vi "find fit -- normalize complex culture.vi"(11 "z in window":cdb[](array[numeric])) -> (0 "z  normalized":cdb[](array[numeric]), 1 "normalization factor":dbl=1.0, 2 "data center":cdb, 3 "# of elements":i32)   [LabVIEW 2021]
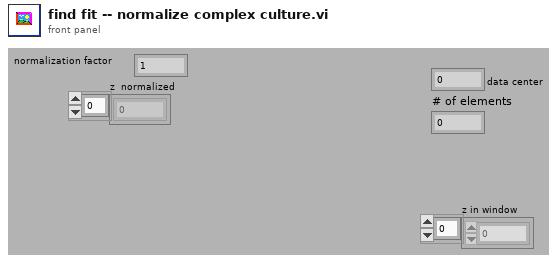
[diagram p1: front panel]
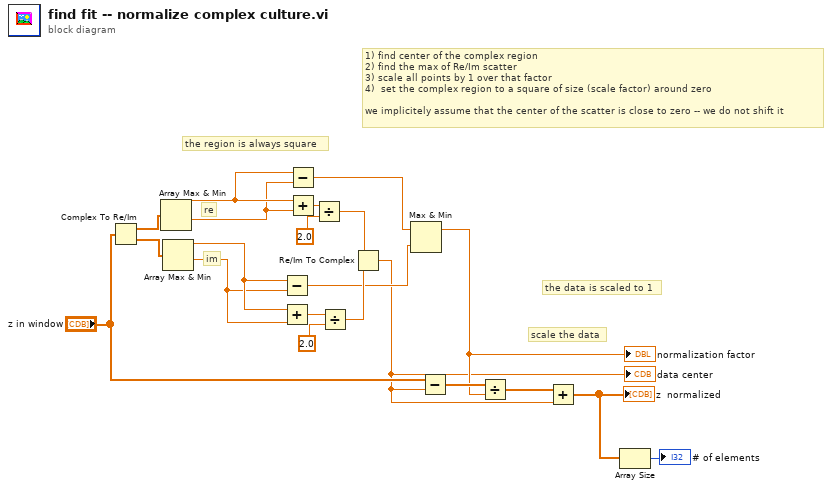
[diagram p0: block diagram]
diagram:
  # "the data is scaled to 1"
  # "scale the data"
  # "1) find center of the complex region\n2) find the max of Re/Im scatter \n3) scale all points by 1 over that factor\n4)  set the complex region to a square of size (scale factor) around zero\n\nwe implicitely assume that the center of the scatter is close to zero -- we do not shift it"
  # "the region is always square"
  # "im"
  # "re"
  n1 = Complex To Re/Im(x + iy="z in window") -> (x=w19:dbl[], y=w18:dbl[])
  n2 = Array Max & Min(array=w19) -> (max value=w14:dbl, min value=w13:dbl)  [unwired: 2 out]
  n3 = Array Max & Min(array=w18) -> (max value=w17:dbl, min value=w16:dbl)  [unwired: 2 out]
  n4 = Subtract(x=w17, y=w16) -> (x-y=w8:dbl)
  n5 = Add(x=w17, y=w16) -> (x+y=w15:dbl)
  n6 = Subtract(x=w14, y=w13) -> (x-y=w9:dbl)
  n7 = Add(x=w14, y=w13) -> (x+y=w12:dbl)
  n8 = Divide(x=w12, y=2.0) -> (x/y=w11:dbl)
  n9 = Divide(x=w15, y=2.0) -> (x/y=w10:dbl)
  n10 = Re/Im To Complex(1:w10, 2:w11) -> (0:w3:cdb)
  "data center" <- w3
  n11 = Max & Min(x=w9, y=w8) -> (max(x,y)=w5:dbl)  [unwired: 1 out]
  "normalization factor" <- w5
  n12 = Subtract(x="z in window", y=w3) -> (x-y=w6:cdb[])
  n13 = Divide(x=w6, y=w5) -> (x/y=w4:cdb[])
  n14 = Add(x=w4, y=w3) -> (x+y=w2:cdb[])
  "z  normalized" <- w2
  n15 = Array Size(array=w2) -> (size(s)=→"# of elements":i32)
